vi "ISEG_HVSystemGUI.constructor.vi"(0 "name":string, 2 "data in":string, 5 "error in (no error)":errorcluster) -> (14 "i ref out":refnum<vi>, 16 "data out":string, 19 "error out":errorcluster)   [LabVIEW 2014, in "ISEG_HVSystemGUI.lvlib"]
doc: "This is the constructor of a class.\n\nLicense Agreement for this software:\n\nCopyright (C)\nGesellschaft für Schwerionenforschung, GSI\nPlanckstr. 1\n64291 Darmstadt\nGermany\n\nContact: D.Beck@gsi.de \n\nThis program is free software; you can redistribute it and/or modify it under the terms of the \nGNU General Public License as published by the Free Software Foundation; either version 2 of \nthe license, or (at your option) any later version.\n\nThis program is distributed in the hope that it will be useful, but WITHOUT ANY WARRANTY; \nwithout even the implied warranty of MERCHANTABILITY or FITNESS FOR A PARTICULAR PURPOSE. See the GNU General License for more details (http://www.gnu.org).\n\nGesellschaft für Schwerionenforschung, GSI\nPlanckstr. 1, 64291 Darmstadt, Germany\nFor all questions and ideas contact: M.Richter@gsi.de, H.Brand@gsi.de or D.Beck@gsi.de.\nLast update: 16-JUN-2004"
uses:
  ISEG_HVSystemGUI.lvlib
  ISEG_HVSystemGUI.i attribute.ctl
  CS_Core/CSObj/CSObj.lvlib
  CS_Core/BaseGUI/BaseGUI.lvlib
  CS_Core/CSSystem/CSSystemLib/CSSystemLib.lvlib
panel:
  in  "CLASS.i attribute":T1
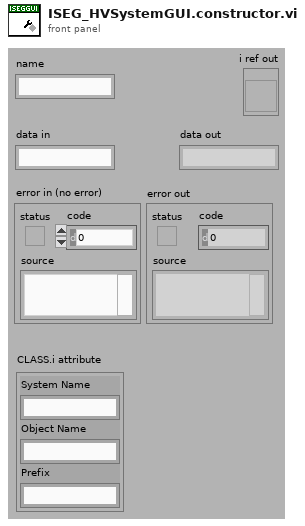
[diagram p1: front panel]
types:
  T1 = typedef "ISEG_HVSystemGUI.lvlib/ISEG_HVSystemGUI.i attribute.ctl" = cluster{"System Name":string, "Object Name":string, "Prefix":string}
  T2 = enum16{"SetAttribute", "GetAttribute", "CreateAttribute", "DestroyAttribute", "DestroyAllAtributes"}
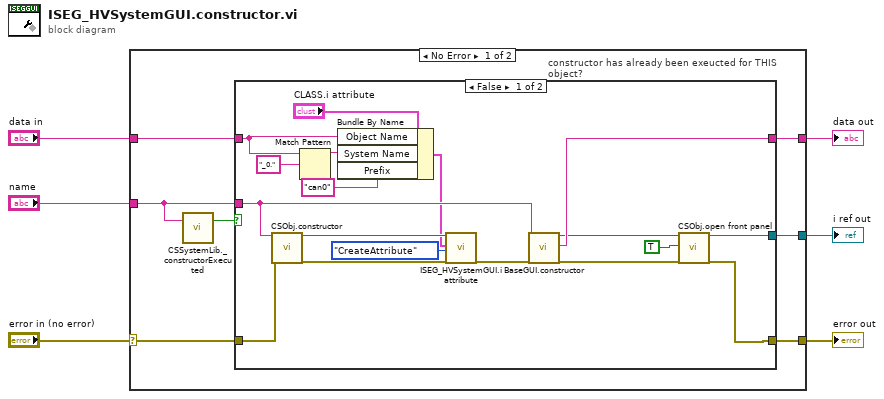
[diagram p0: block diagram]
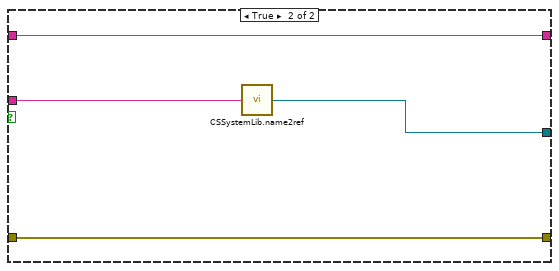
[diagram p2: hidden frame]
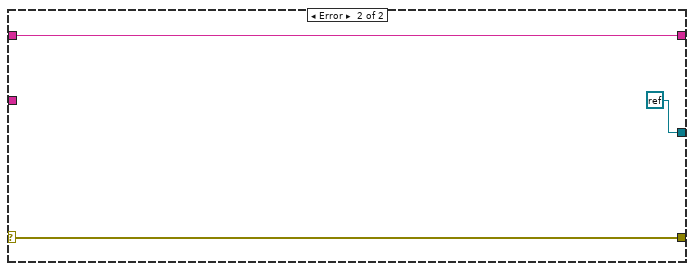
[diagram p3: hidden frame]
diagram:
  n1 = case shown="No Error" "error in (no error)" {
    selector: "error in (no error)" -> [w10 w37]
    tunnel: "data in" -> [w13 w36]
    tunnel: "name" -> [w9 _]
    tunnel: [w12 refnum<k0> refnum] -> w4
    tunnel: [w11 w37] -> w3
    tunnel: [w7 w36] -> w1
    frame No Error {
      n2 = call "CSSystemLib._constructorExecuted.vi"("name"=w9) -> ("constructor executed?"=w8:bool)  [unwired: 18 in]
      n3 = case "constructor has already been exeucted for THIS object?" shown="False" w8 {
        tunnel: w13 -> [w22 w32]
        tunnel: w9 -> [w28 w35]
        tunnel: [w15 w34] -> w12
        tunnel: [w17 w33] -> w11
        tunnel: w10 -> [w26 w33]
        tunnel: [w25 w32] -> w7
        frame False {
          n4 = call "CSObj.constructor.vi"("name"=w28, "error in (no error)"=w26) -> ("i ref out"=w30:refnum<vi>, "error out"=w29:errorcluster)  [unwired: 15 in, 1 out]
          n5 = Match Pattern(string=w22, regular expression="_0.") -> (before substring=w21:string)  [unwired: 1 in, 3 out]
          n6 = Bundle By Name(cluster="CLASS.i attribute", "Object Name"=w22, "System Name"=w21, "Prefix"="can0") -> (w20:T1)
          n7 = call "ISEG_HVSystemGUI.i attribute.vi"("VI Refnum"=w30, "CLASS.i attribute"=w20, "Action"=T2."CreateAttribute", "error in (no error)"=w29) -> ("error out"=w27:errorcluster)  [unwired: 13 in, 2 out]
          n8 = call "BaseGUI.constructor.vi"("name"=w28, "error in (no error)"=w27) -> ("i ref out"=w16:refnum<vi>, "data out"=w25:string, "error out"=w18:errorcluster)  [unwired: 15 in]
          n9 = call "CSObj.open front panel.vi"("i ref in"=w16, "frontPanelOpen"=TRUE ("front panel open"), "error in (no error)"=w18) -> ("i ref out"=w15:refnum<vi>, "error out"=w17:errorcluster)  [unwired: 15 in]
        }
        frame True {
          n10 = call "CSSystemLib.name2ref.vi"("name"=w35) -> ("obj refnum"=w34:refnum<vi>)
        }
      }
    }
    frame Error {
    }
  }
  "i ref out" <- w4
  "error out" <- w3
  "data out" <- w1
